vi "main_VI.vi"() -> ()   [LabVIEW 2013]
panel:
  in  "stop":bool
  out "100 punti letti":dbl[](graph)
  in  "start acqusition":bool
  in  "ampiezza":dbl
  in  "tipo":enum16{"sin", "squ", "tri"}(ring)
  in  "frequenza":dbl
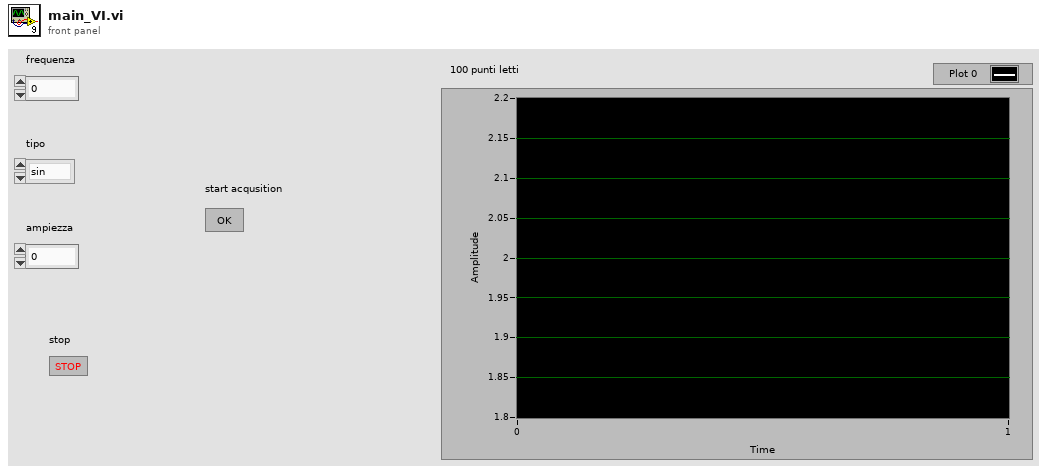
[diagram p1: front panel]
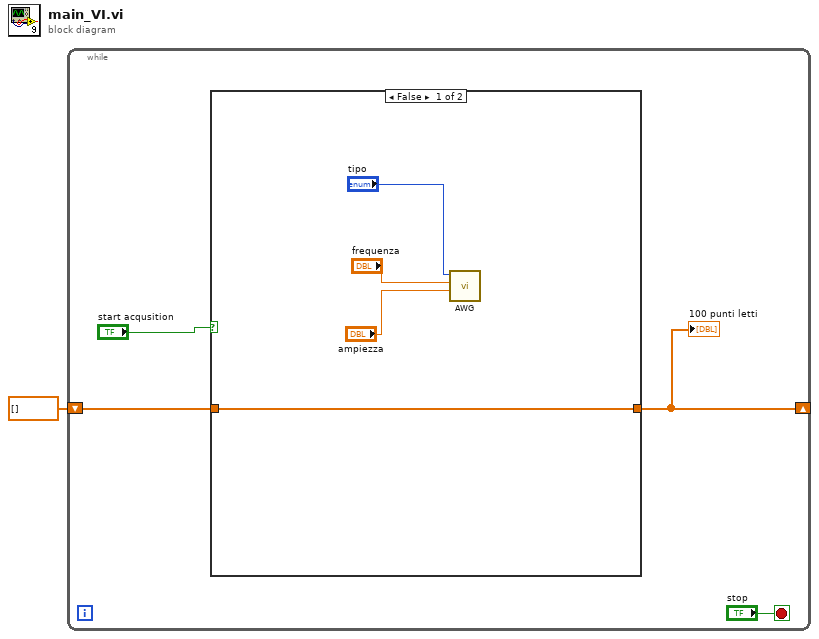
[diagram p0: block diagram]
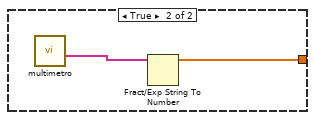
[diagram p2: hidden frame]
diagram:
  n1 = while {
    shift-right: [w3] -> _
    shift-left: dbl[] [] -> [w2]
    stop <- "stop" stop-if-true
    n2 = case shown="False" "start acqusition" {
      tunnel: [w9 w10] -> w3
      tunnel: w2 -> [w9 _]
      frame False {
        n3 = call "AWG.vi"("ampiezza"="ampiezza", "frequenza"="frequenza", "tipo"="tipo") -> ()  [unwired: 9 in]
      }
      frame True {
        n4 = call "multimetro.vi"() -> ("100 misure"=w11:string[])  [unwired: 11 in]
        n5 = Fract/Exp String To Number(string=w11) -> (number=w10:dbl[])  [unwired: 3 in, 1 out]
      }
    }
    "100 punti letti" <- w3
  }
